vi "Configure.vi"(8 "error in (no error)":errorcluster, 11 "Template in":refnum<class "Cobolt.lvclass">) -> (0 "error out":errorcluster={"status"=TRUE, "code"=-8001, "source"="Failed to set autostart state on laser! Port: Com9 \n\nNo response from Laser!\n \nMake sure it is powered on and properly connected to the PC.\n\nExpected minimum length response format: 2 non-digit(s)\n\nCall chain: Cobolt.lvclass:CoboltLaser_ResponseCheck.viCobolt.lvclass:VISA response check.viCobolt.lvclass:VISA.viCobolt.lvclass:set autostart enable status.viCobolt.lvclass:Configure.viMurmex.lvlib:Murmex.lvclass:Initialise.viCobolt.lvclass:Initialise.viMurmex.lvlib:Murmex.lvclass:Handle messages.vi:1Cobolt.lvclass:Main.vi"}, 2 "cancelled?":bool, 3 "Template out":refnum<class "Cobolt.lvclass">)   [LabVIEW 2012, in "Cobolt.lvclass"]
doc: "The configure method configures the details for the RabbitMQ connection. \n\nIn the derived class, make a call to the parent for setting these parameters."
uses:
  Cobolt.lvclass
  laser lines.ctl
  <vilib>/Utility/miscctls.llb/LVPointTypeDef.ctl
  Cobolt.lvclass/Cobolt.ctl
  <vilib>/Distrio/Murmex/Murmex/Murmex.lvclass
panel:
  in  "Tab Control":enum32{"Comport", "Debug"}(tab)
  in  "Generate Error if Fail":bool=TRUE
  in  "Laser line":T1=9 items=["405nm"=4, "445nm"=6, "491nm"=8, "515nm"=9, "561nm"=10]
  in  "Autostart":bool
  in  "VISA Wait":dbl[unit]=0.5
  in  "Enable Term Char":u16(ring) items=["Off", "On"]
  in  "Baud rate":u32=115200
  in  "parity":u16(ring) items=["None", "Odd", "Even", "Mark", "Space"]
  in  "stop bits":u16(ring)=10 items=["1.0"=10, "1.5"=15, "2.0"=20]
  in  "Flow control":u16(ring) items=["None"=0, "XON/XOFF"=1, "RTS/CTS"=2, "DTR/DSR"=4]
  in  "data bits":u16=8 min=5 max=8 step=1
  in  "Time out":u32=3000
  in  "Key switch state":bool=TRUE
  in  "button:call parent":bool
  in  "button:ok":bool
  in  "button:cancel":bool
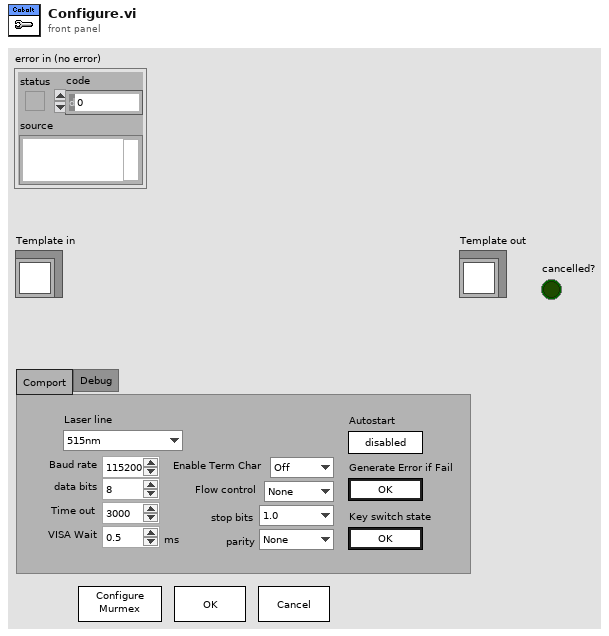
[diagram p1: front panel]
types:
  T1 = typedef "Cobolt.lvclass/laser lines.ctl" = u16
  T2 = typedef "LVPointTypeDef.ctl" = cluster{"Horizontal":i16, "Vertical":i16}
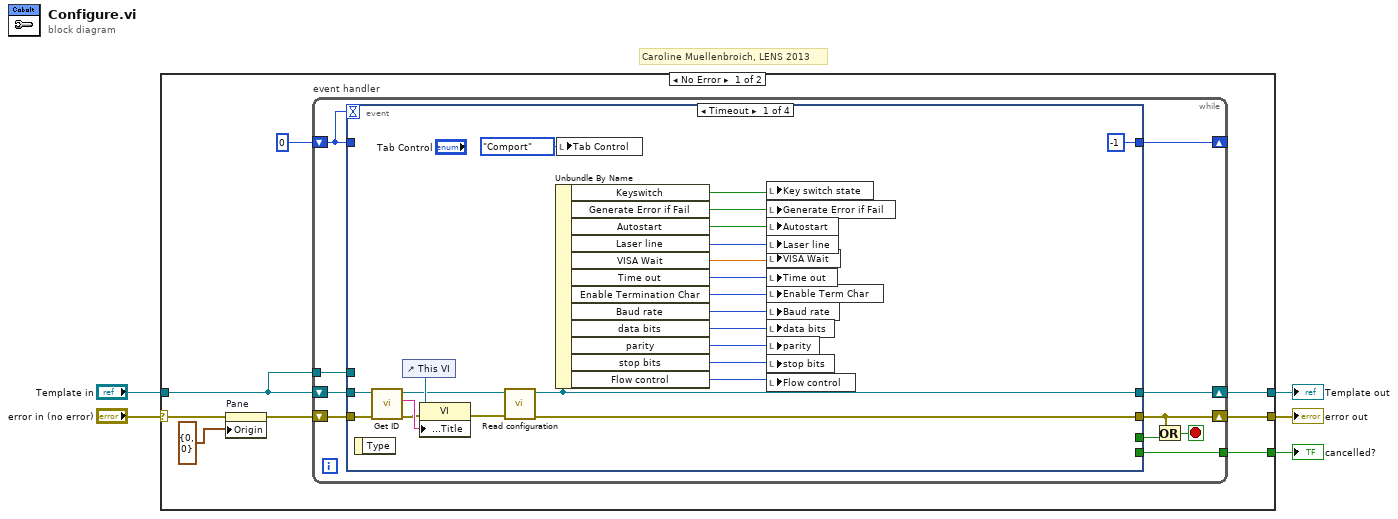
[diagram p0: block diagram]
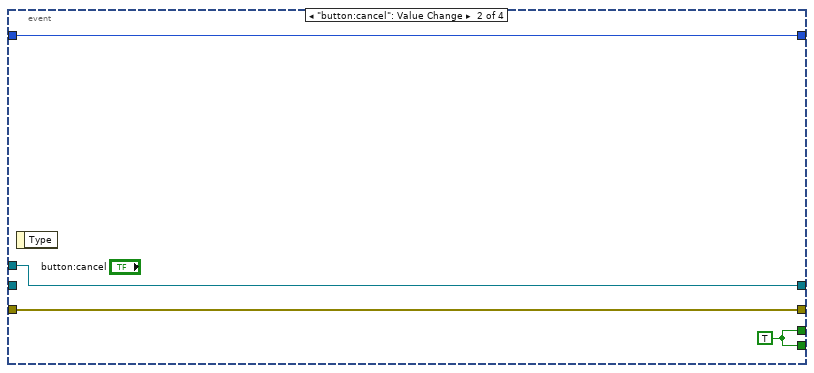
[diagram p2: hidden frame]
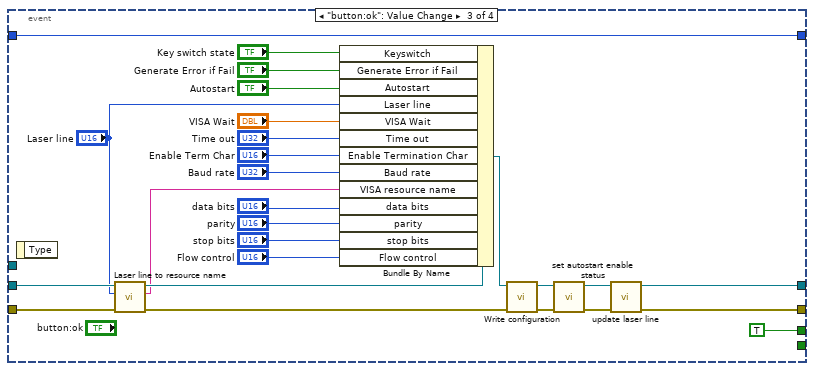
[diagram p3: hidden frame]
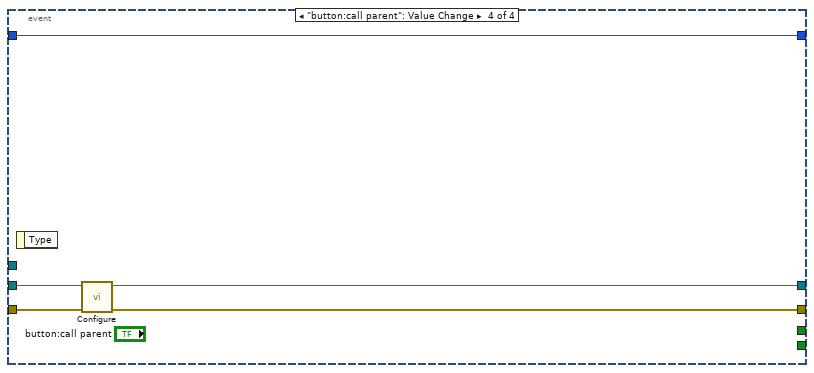
[diagram p4: hidden frame]
diagram:
  # "Caroline Muellenbroich, LENS 2013"
  n1 = case shown="No Error" "error in (no error)" {
    selector: "error in (no error)" -> [w11 w83]
    tunnel: "Template in" -> [w9 w82]
    tunnel: [w8 w82] -> w3
    tunnel: [w7 w83] -> w2
    tunnel: [w6 _] -> w1
    frame No Error {
      n2 = property on="Pane" class="Pane"(error in=w11, "Origin"=T2 {"Horizontal"=0, "Vertical"=0}) -> (error out=w10:errorcluster)  [unwired: 1 in, 1 out]
      n3 = while "event handler" {
        tunnel: [w23] -> w6
        shift-right: [w22] -> w8
        shift-left: w9 -> [w15]
        shift-right: [w20] -> w7
        shift-left: w10 -> [w21]
        shift-right: [w14] -> _
        shift-left: 0 -> [w17]
        tunnel: w9 -> [w16]
        stop <- w18 stop-if-true
        n4 = event shown="[0] Timeout" {
          selector: _ -> [_ _ _ _]
          dyn-events: _ -> [_ _ _ _]
          timeout: w17 -> [_ _ _ _]
          tunnel: [w46 w49 w54 w79] -> w20
          tunnel: [_ w48 _ _] -> w23
          tunnel: [w45 w50 w55 w78] -> w22
          tunnel: w21 -> [w40 w49 w65 w80]
          tunnel: w15 -> [w39 _ w64 w81]
          tunnel: w16 -> [_ w50 _ _]
          tunnel: [_ w48 TRUE ("cancelled?") _] -> w19
          tunnel: w17 -> [_ w47 w74 w77]
          tunnel: [-1 w47 w74 w77] -> w14
          event Timeout {
            n5 = event-data() -> ()  [unwired: 1 in, 1 out]
            n6 = call <vilib>:"Get ID.vi"("error in (no error)"=w40, "Murmex in"=w39) -> ("error out"=w42:errorcluster, "component id"=w43:string, "Murmex out"=w38:refnum<class "Cobolt.lvclass">)  [unwired: 7 in]
            n7 = control-ref of="This VI"() -> (w41:refnum<vi>)
            n8 = property class="VI"(reference=w41, error in=w42, "Front Panel.Title"=w43) -> (error out=w37:errorcluster)  [unwired: 1 out]
            n9 = call <vilib>:"Read configuration.vi"("error in (no error)"=w37, "Murmex in"=w38) -> ("error out"=w46:errorcluster, "Murmex out"=w45:refnum<class "Cobolt.lvclass">)  [unwired: 7 in, 1 out]
            n10 = Unbundle By Name(w45) -> ("Keyswitch"=w24:bool, "Generate Error if Fail"=w25:bool, "Autostart"=w26:bool, "Laser line"=w27:T1, "VISA Wait"=w35:dbl[unit], "Time out"=w34:u32, "Enable Termination Char"=w33:u16, "Baud rate"=w32:u32, "data bits"=w31:u16, "parity"=w30:u16, "stop bits"=w29:u16, "Flow control"=w28:u16)
            n11 = local write "Tab Control"(enum32{"Comport", "Debug"}."Comport" ("Tab Control")) -> ()
            n12 = local write "Key switch state"(w24) -> ()
            n13 = local write "Generate Error if Fail"(w25) -> ()
            n14 = local write "Autostart"(w26) -> ()
            n15 = local write "Laser line"(w27) -> ()
            n16 = local write "VISA Wait"(w35) -> ()
            n17 = local write "Time out"(w34) -> ()
            n18 = local write "Enable Term Char"(w33) -> ()
            n19 = local write "Baud rate"(w32) -> ()
            n20 = local write "data bits"(w31) -> ()
            n21 = local write "parity"(w30) -> ()
            n22 = local write "stop bits"(w29) -> ()
            n23 = local write "Flow control"(w28) -> ()
          }
          event "button:cancel": Value Change {
            w48 = TRUE ("cancelled?")
            n24 = event-data() -> ()  [unwired: 1 in, 1 out]
          }
          event "button:ok": Value Change {
            n25 = event-data() -> ()  [unwired: 1 in, 1 out]
            n26 = call-dynamic "Laser line to resource name.vi"("error in (no error)"=w65, "Laser line"="Laser line", "Cobolt in"=w64) -> ("error out"=w62:errorcluster, "VISA resource"=w61:string, "Cobolt out"=w63:refnum<class "Cobolt.lvclass">)  [unwired: 6 in]
            n27 = Bundle By Name(cluster=w63, "Keyswitch"="Key switch state", "Generate Error if Fail"="Generate Error if Fail", "Autostart"="Autostart", "Laser line"="Laser line", "VISA Wait"="VISA Wait", "Time out"="Time out", "Enable Termination Char"="Enable Term Char", "Baud rate"="Baud rate", "VISA resource name"=w61, "data bits"="data bits", "parity"="parity", "stop bits"="stop bits", "Flow control"="Flow control") -> (w75:refnum<class "Cobolt.lvclass">)
            n28 = call <vilib>:"Write configuration.vi"("error in (no error)"=w62, "Murmex in"=w75) -> ("error out"=w59:errorcluster, "Murmex out"=w58:refnum<class "Cobolt.lvclass">)  [unwired: 8 in]
            n29 = call-dynamic "set autostart enable status.vi"("error in (no error)"=w59, "Cobolt in"=w58) -> ("error out"=w57:errorcluster, "Cobolt out"=w56:refnum<class "Cobolt.lvclass">)  [unwired: 8 in]
            n30 = call-dynamic "update laser line.vi"("error in (no error)"=w57, "Cobolt in"=w56) -> ("error out"=w54:errorcluster, "Cobolt out"=w55:refnum<class "Cobolt.lvclass">)  [unwired: 8 in]
          }
          event "button:call parent": Value Change {
            n31 = event-data() -> ()  [unwired: 1 in, 1 out]
            n32 = call-parent "Configure.vi"("error in (no error)"=w80, "Murmex in"=w81) -> ("error out"=w79:errorcluster, "Murmex out"=w78:refnum<class "Cobolt.lvclass">)  [unwired: 7 in, 1 out]
          }
        }
        n33 = Or(x=w20, y=w19) -> (x .or. y?=w18:bool)
      }
    }
    frame Error {
    }
  }
  "error out" <- w2
  "Template out" <- w3
  "cancelled?" <- w1
